vi "Tree_MouseUp position.vi"(0 "CtlRef in":refnum<vi>, 7 "Coords":T1, 11 "error in (no error)":errorcluster) -> (4 "dup CtlRef":refnum<vi>, 6 "Col":i32, 8 "Tag":string, 13 "InSymbol":bool, 14 "InBounds":bool, 15 "error out":errorcluster)   [LabVIEW 2014]
uses:
  <vilib>/Utility/miscctls.llb/LVPositionTypeDef.ctl
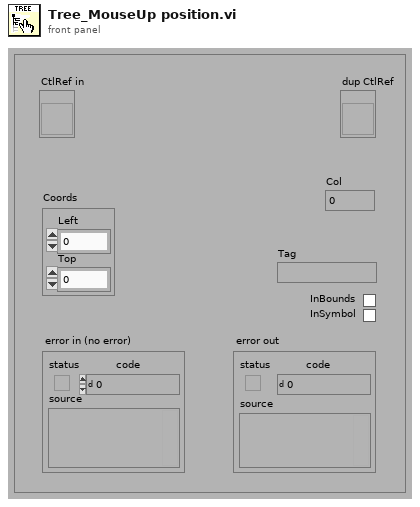
[diagram p1: front panel]
types:
  T1 = typedef "LVPositionTypeDef.ctl" = cluster{"Left":i32, "Top":i32}
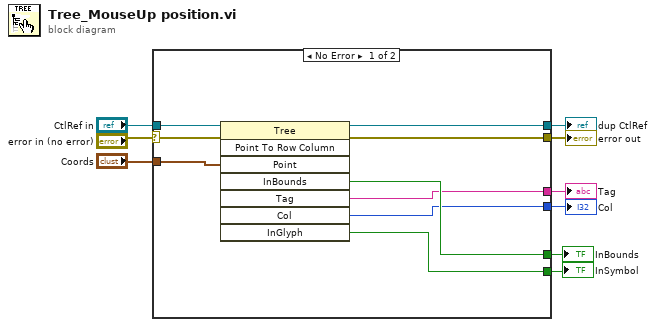
[diagram p0: block diagram]
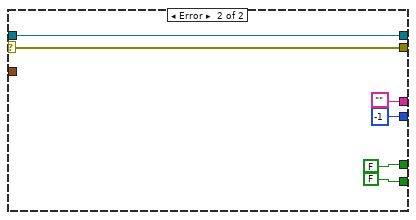
[diagram p2: hidden frame]
diagram:
  n1 = case shown="No Error" "error in (no error)" {
    selector: "error in (no error)" -> [w16 w24]
    tunnel: "CtlRef in" -> [w17 w23]
    tunnel: "Coords" -> [w18 _]
    tunnel: [w11 w23] -> w4
    tunnel: [w13 -1 ("Col")] -> w1
    tunnel: [w12 ""] -> w2
    tunnel: [w15 FALSE ("InBounds")] -> w6
    tunnel: [w14 FALSE ("InGlyph")] -> w3
    tunnel: [w10 w24] -> w5
    frame No Error {
      n2 = invoke class="Tree" method="Point To Row Column"(reference=w17, error in=w16, "Point"=w18) -> (reference out=w11:refnum<vi>, error out=w10:errorcluster, "InBounds"=w15:bool, "Tag"=w12:string, "Col"=w13:i32, "InGlyph"=w14:bool)  [unwired: 5 in, 2 out]
    }
    frame Error {
    }
  }
  "InBounds" <- w6
  "error out" <- w5
  "dup CtlRef" <- w4
  "InSymbol" <- w3
  "Tag" <- w2
  "Col" <- w1
